vi "GLVT-Main_SingleLoop.vi"() -> ()   [LabVIEW 2020]
uses:
  Controls/GLVT-Stepper-EnableState.ctl
  Controls/GLVT-FlowmeterBankSelection.ctl
  Controls/GLVT-States.ctl
  Controls/GLVT-FGV-States.ctl
  Controls/GLVT-Stepper-RotateDirection.ctl
panel:
  in  "Flowmeter Bank":T1
  in  "Data Measure Time":dbl=1.0 min=1.0 step=0.1 format="%<%H:%M:%S>t"
  in  "Stop Button":bool
  out "Filename DTS":string
  out "Save Data Location":path
  in  "Filename Descriptor":string
  out "End Data Collection":bool
  out "Current Angle Array Location":i32
  out "Working":bool
  in  "Measure Valve Button":bool
  out "Collected Data":cluster{dbl[], dbl[]}(graph)
  out "Angles for Data Collection (deg abs)":dbl[](array[numeric])
  in  "Angle per Step":dbl=1.0 min=1.0 step=0.1
  in  "Max Angle to Rotate (deg abs)":dbl
  in  "Pulse Rate (pps)":i32=600
  in  "Steps per Rev":i32=1600
  in  "Move Stepper Button":bool
  in  "Angle to Rotate  (deg abs)":dbl step=0.1
  out "Motor Position Actual":dbl format="%#.2f"
  in  "Release Motor Button":bool
  in  "Motor State":T2
  # "Configuration Only\nDo Not Change"
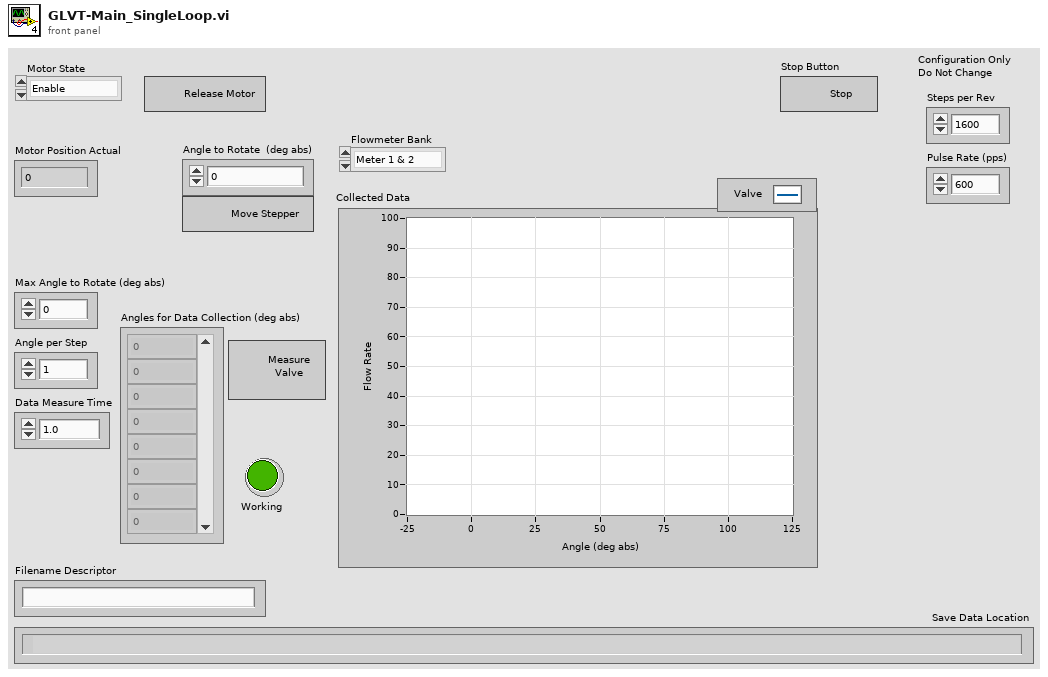
[diagram p1: front panel]
types:
  T1 = typedef "GLVT-FlowmeterBankSelection.ctl" = enum16{"Meter 1 & 2", "Meter 3 & 4", "Meter 5 & 6"}
  T2 = typedef "GLVT-Stepper-EnableState.ctl" = enum16{"Enable", "Disable"}
  T3 = typedef "GLVT-States.ctl" = enum16{"Idle", "Initialize", "Read Data", "Next Valve Pos", "Rotate Valve", "Save Data", "Exit"}
  T4 = typedef "GLVT-FGV-States.ctl" = enum16{"Get", "Set"}
  T5 = typedef "GLVT-Stepper-RotateDirection.ctl" = enum16{"CCW", "CW"}
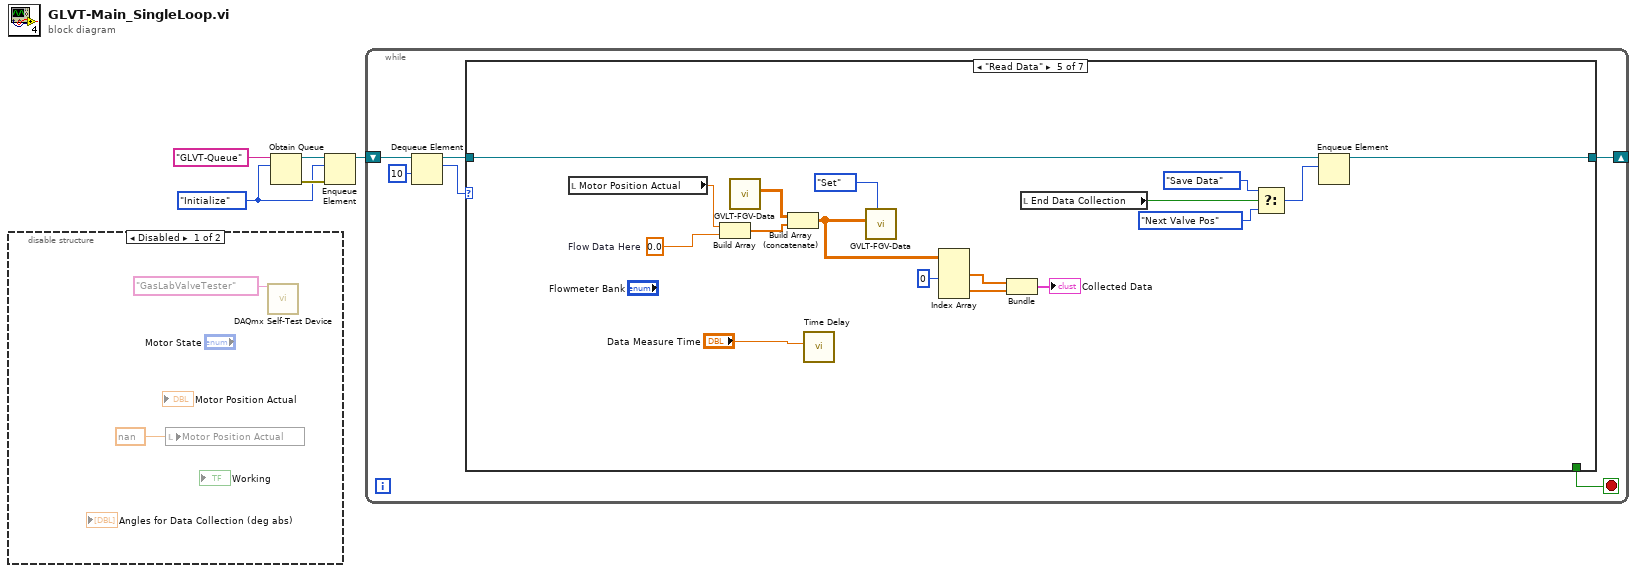
[diagram p0: block diagram]
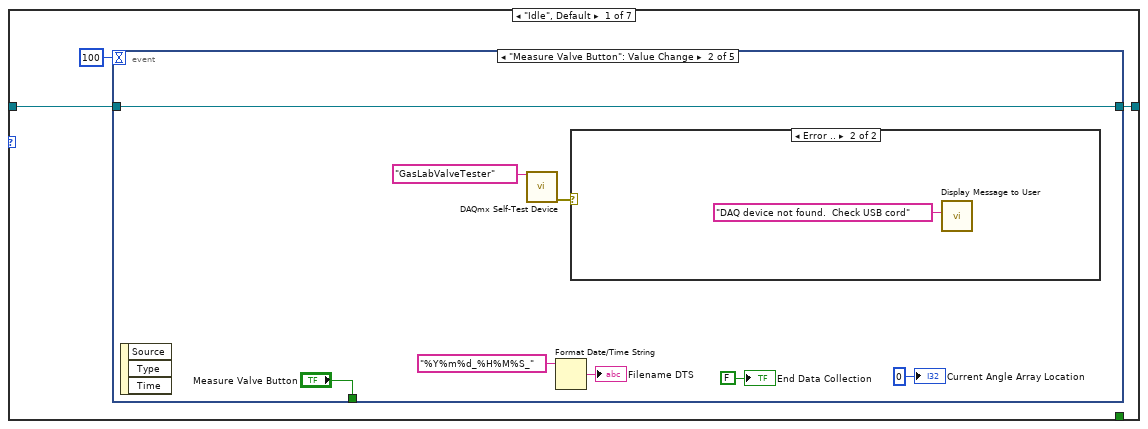
[diagram p2: hidden frame]
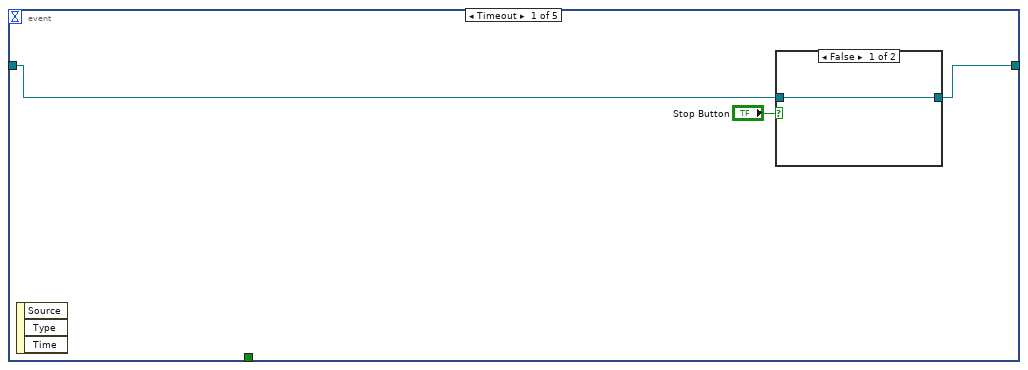
[diagram p3: hidden frame]
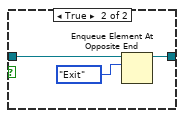
[diagram p4: hidden frame]
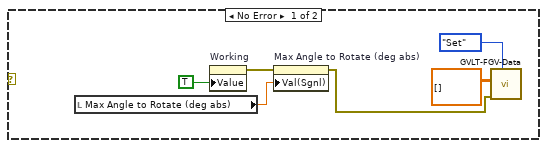
[diagram p5: hidden frame]
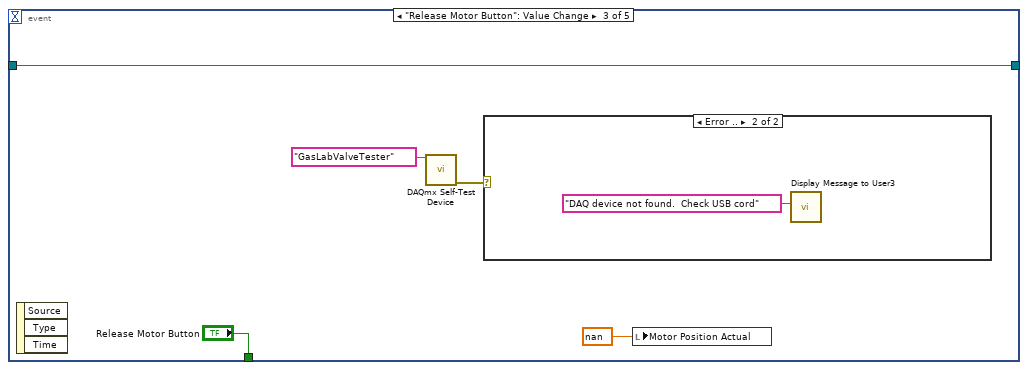
[diagram p6: hidden frame]
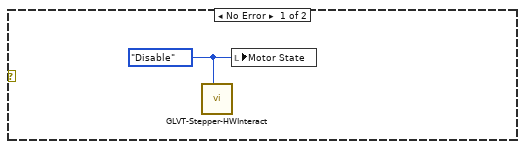
[diagram p7: hidden frame]
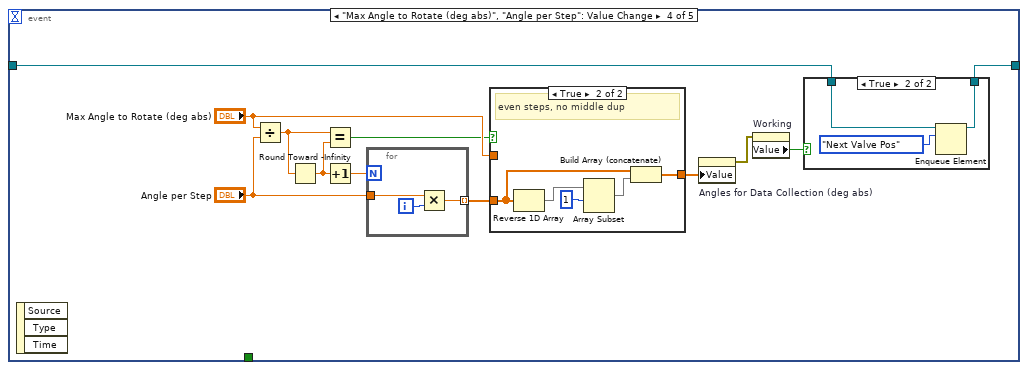
[diagram p8: hidden frame]
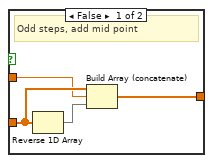
[diagram p10: hidden frame]
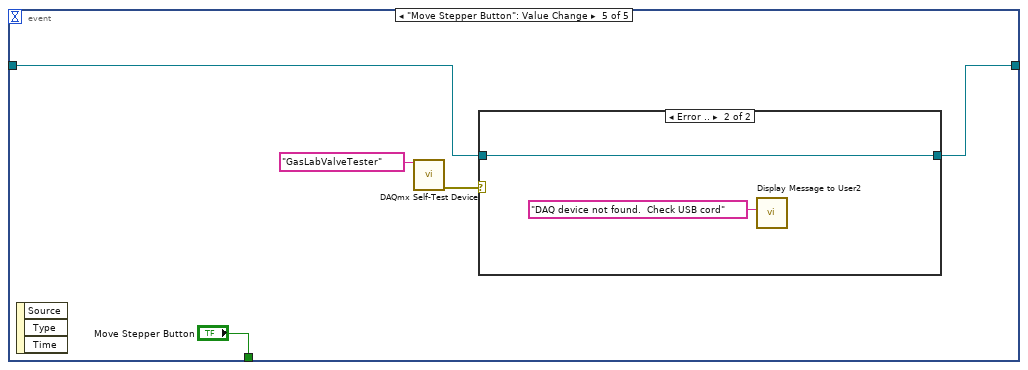
[diagram p11: hidden frame]
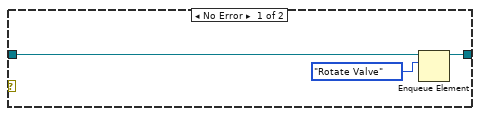
[diagram p12: hidden frame]
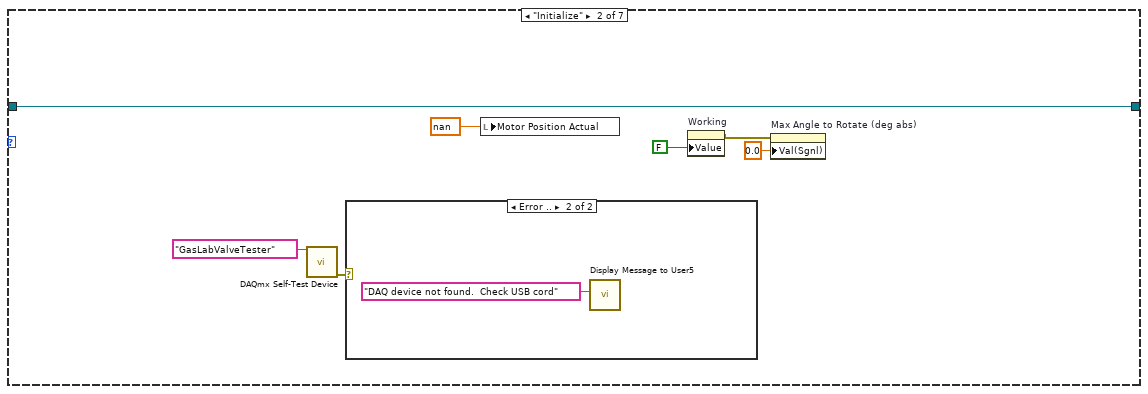
[diagram p13: hidden frame]
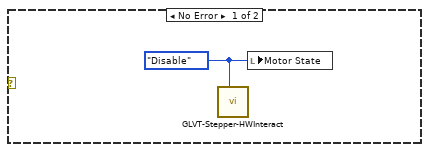
[diagram p14: hidden frame]
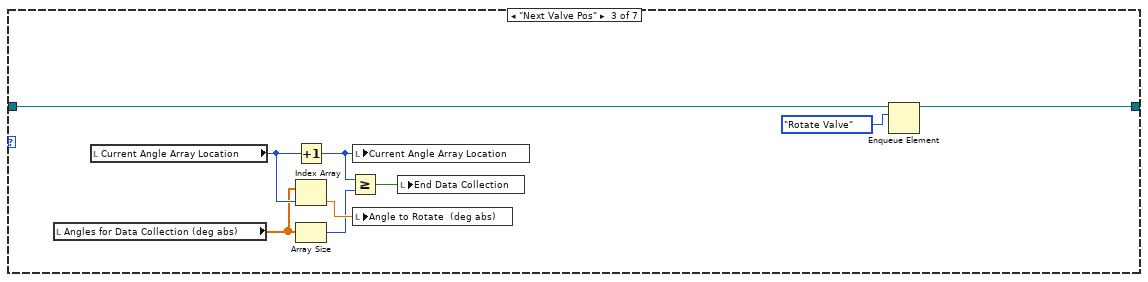
[diagram p15: hidden frame]
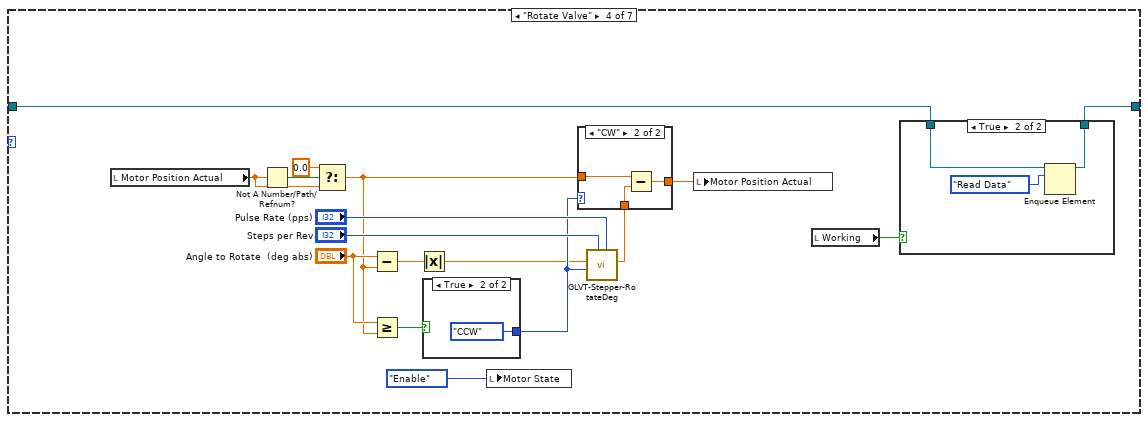
[diagram p16: hidden frame]
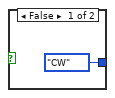
[diagram p18: hidden frame]
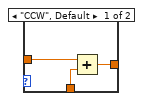
[diagram p19: hidden frame]
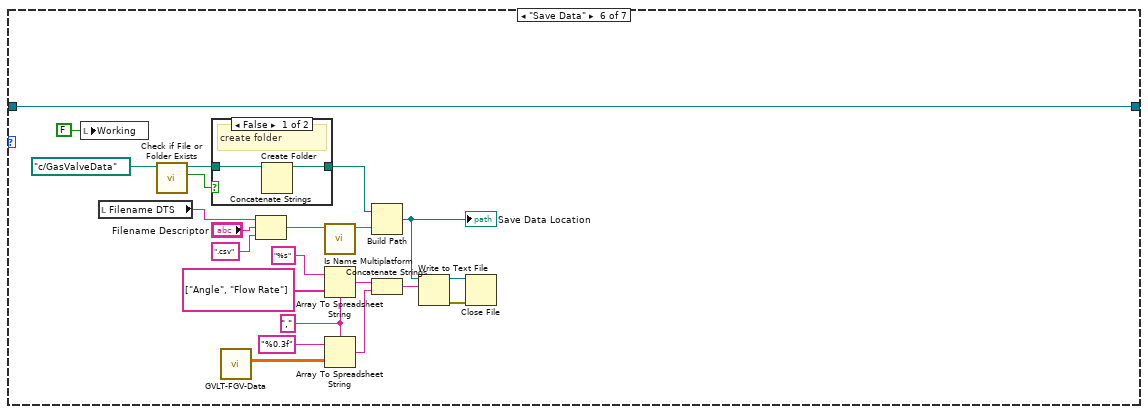
[diagram p20: hidden frame]
diagram:
  w2 = GLVT-States."Initialize"
  n1 = disable-structure shown="Disabled" {
    frame Disabled {
      n2 = local write "Motor Position Actual"(nan ("Motor Position")) -> ()
      n3 = call <vilib>:"DAQmx Self-Test Device.vi"("device in"=tag "GasLabValveTester") -> ()  [unwired: 14 in, 1 out]
    }
    frame Enabled {
    }
  }
  n4 = Obtain Queue(name (unnamed)="GLVT-Queue", element data type=w2) -> (queue out=w3:refnum<queue>, error out=w4:errorcluster)  [unwired: 3 in, 1 out]
  n5 = Enqueue Element(queue=w3, element=w2, error in (no error)=w4) -> (queue out=w1:refnum<queue>)  [unwired: 1 in, 2 out]
  n6 = while {
    shift-right: [w9] -> _
    shift-left: w1 -> [w12]
    stop <- w13 stop-if-true
    n7 = Dequeue Element(queue=w12, timeout in ms (-1)=10) -> (queue out=w11:refnum<queue>, element=w10:T3)  [unwired: 1 in, 2 out]
    n8 = case shown="\"Read Data\"" w10 {
      tunnel: [_ _ _ _ _ _ TRUE] -> w13
      tunnel: w11 -> [w15 w90 w101 w103 w147 w169 w177]
      tunnel: [w14 w90 w94 w102 w146 w169 w177] -> w9
      frame "Idle", Default {
        n9 = event shown="[1] \"Measure Valve Button\": Value Change" {
          selector: _ -> [_ _ _ _ _]
          dyn-events: _ -> [_ _ _ _ _]
          timeout: 100 -> [_ _ _ _ _]
          tunnel: w15 -> [w18 w31 w43 w47 w78]
          tunnel: [w19 w31 w43 w46 w76] -> w14
          tunnel: [_ "Measure Valve Button" "Release Motor Button" _ "Move Stepper Button"] -> _
          event Timeout {
            n10 = event-data() -> ()  [unwired: 1 in, 3 out]
            n11 = case shown="False" "Stop Button" {
              tunnel: [w20 w22] -> w19
              tunnel: w18 -> [w20 w21]
              frame False {
              }
              frame True {
                n12 = Enqueue Element At Opposite End(queue=w21, element=GLVT-States."Exit") -> (queue out=w22:refnum<queue>)  [unwired: 2 in, 2 out]
              }
            }
          }
          event "Measure Valve Button": Value Change {
            n13 = event-data() -> ()  [unwired: 1 in, 3 out]
            n14 = call <vilib>:"DAQmx Self-Test Device.vi"("device in"=tag "GasLabValveTester") -> ("error out"=w24:errorcluster)  [unwired: 14 in]
            n15 = Format Date/Time String(time format string (%c)="%Y%m%d_%H%M%S_") -> (date/time string=→"Filename DTS":string)  [unwired: 2 in]
            n16 = case shown="Error .." w24 {
              frame No Error {
                n17 = local read "Max Angle to Rotate (deg abs)"() -> (w37:dbl)
                n18 = property on="Working" class="Bool (strict)"("Value"=TRUE ("Working")) -> (error out=w35:errorcluster)  [unwired: 2 in, 1 out]
                n19 = property on="Max Angle to Rotate (deg abs)" class="DigNum (strict)"(error in=w35, "Val(Sgnl)"=w37) -> (error out=w32:errorcluster)  [unwired: 1 in, 1 out]
                n20 = call "GVLT-FGV-Data.vi"("State"=GLVT-FGV-States."Set", "error in"=w32, "Data In"=dbl[][] []) -> ()  [unwired: 7 in, 2 out]
              }
              frame Error {
                n21 = call "Display Message to User"("Message"="DAQ device not found.  Check USB cord") -> ()  [unwired: 9 in, 2 out]
              }
            }
            "Current Angle Array Location" <- 0 ("Current Angle Array Location")
            "End Data Collection" <- FALSE ("End Data Collection")
          }
          event "Release Motor Button": Value Change {
            n22 = event-data() -> ()  [unwired: 1 in, 3 out]
            n23 = call <vilib>:"DAQmx Self-Test Device.vi"("device in"=tag "GasLabValveTester") -> ("error out"=w39:errorcluster)  [unwired: 14 in]
            n24 = case shown="Error .." w39 {
              frame No Error {
                w44 = GLVT-Stepper-EnableState."Disable" ("GLVT-Enable State")
                n25 = call "GLVT-Stepper-HWInteract.vi"("GLVT-Enable State"=w44) -> ()  [unwired: 10 in, 1 out]
                n26 = local write "Motor State"(w44) -> ()
              }
              frame Error {
                n27 = call "Display Message to User3"("Message"="DAQ device not found.  Check USB cord") -> ()  [unwired: 9 in, 2 out]
              }
            }
            n28 = local write "Motor Position Actual"(nan ("Motor Position")) -> ()
          }
          event "Max Angle to Rotate (deg abs)", "Angle per Step": Value Change {
            n29 = event-data() -> ()  [unwired: 1 in, 3 out]
            n30 = Divide(x="Max Angle to Rotate (deg abs)", y="Angle per Step") -> (x/y=w53:dbl)
            n31 = Round Toward -Infinity(1:w53) -> (0:w52:dbl)
            n32 = Equal?(x=w53, y=w52) -> (x = y?=w51:bool)
            n33 = Increment(x=w52) -> (x+1=w57:dbl)
            n34 = for {
              N: w57 -> [_]
              tunnel: "Angle per Step" -> [w72]
              tunnel: [w71] -> w55 mode=indexing
              i -> [w73]
              n35 = Multiply(x=w72, y=w73) -> (x*y=w71:dbl)
            }
            n36 = case shown="True" w51 {
              tunnel: [w65 w66] -> w50
              tunnel: w55 -> [w64 w67]
              tunnel: "Max Angle to Rotate (deg abs)" -> [w62 _]
              frame False {
                # "Odd steps, add mid point"
                n37 = Reverse 1D Array(array=w64) -> (reversed array=w63:dbl[])
                n38 = Build Array (concatenate)(w64, w62, w63) -> (w65:dbl[])
              }
              frame True {
                # "even steps, no middle dup"
                n39 = Reverse 1D Array(array=w67) -> (reversed array=w70:dbl[])
                n40 = Array Subset(array=w70, index=1) -> (w68:dbl[])  [unwired: 1 in]
                n41 = Build Array (concatenate)(w67, w68) -> (w66:dbl[])
              }
            }
            n42 = property on="Angles for Data Collection (deg abs)" class="Arr (strict)"("Value"=w50) -> (error out=w49:errorcluster)  [unwired: 2 in, 1 out]
            n43 = property on="Working" class="Bool (strict)"(error in=w49) -> ("Value"=w48:bool)  [unwired: 1 in, 2 out]
            n44 = case shown="True" w48 {
              tunnel: [w58 w60] -> w46
              tunnel: w47 -> [w58 w61]
              frame False {
              }
              frame True {
                n45 = Enqueue Element(queue=w61, element=GLVT-States."Next Valve Pos") -> (queue out=w60:refnum<queue>)  [unwired: 2 in, 2 out]
              }
            }
          }
          event "Move Stepper Button": Value Change {
            n46 = event-data() -> ()  [unwired: 1 in, 3 out]
            n47 = call <vilib>:"DAQmx Self-Test Device.vi"("device in"=tag "GasLabValveTester") -> ("error out"=w74:errorcluster)  [unwired: 14 in]
            n48 = case shown="Error .." w74 {
              tunnel: w78 -> [w81 w83]
              tunnel: [w80 w83] -> w76
              frame No Error {
                n49 = Enqueue Element(queue=w81, element=GLVT-States."Rotate Valve") -> (queue out=w80:refnum<queue>)  [unwired: 2 in, 2 out]
              }
              frame Error {
                n50 = call "Display Message to User2"("Message"="DAQ device not found.  Check USB cord") -> ()  [unwired: 9 in, 2 out]
              }
            }
          }
        }
      }
      frame "Initialize" {
        n51 = call <vilib>:"DAQmx Self-Test Device.vi"("device in"=tag "GasLabValveTester") -> ("error out"=w84:errorcluster)  [unwired: 14 in]
        n52 = case shown="Error .." w84 {
          frame No Error {
            w91 = GLVT-Stepper-EnableState."Disable" ("GLVT-Enable State")
            n53 = call "GLVT-Stepper-HWInteract.vi"("GLVT-Enable State"=w91) -> ()  [unwired: 10 in, 1 out]
            n54 = local write "Motor State"(w91) -> ()
          }
          frame Error {
            n55 = call "Display Message to User5"("Message"="DAQ device not found.  Check USB cord") -> ()  [unwired: 9 in, 2 out]
          }
        }
        n56 = local write "Motor Position Actual"(nan ("Motor Position")) -> ()
        n57 = property on="Working" class="Bool (strict)"("Value"=FALSE ("Working")) -> (error out=w86:errorcluster)  [unwired: 2 in, 1 out]
        n58 = property on="Max Angle to Rotate (deg abs)" class="DigNum (strict)"(error in=w86, "Val(Sgnl)"=0.0 ("Value (Signaling)")) -> ()  [unwired: 1 in, 2 out]
      }
      frame "Next Valve Pos" {
        n59 = local read "Angles for Data Collection (deg abs)"() -> (w98:dbl[])
        n60 = local read "Current Angle Array Location"() -> (w100:i32)
        n61 = Increment(x=w100) -> (x+1=w96:i32)
        n62 = Index Array(array=w98, index=w100) -> (element=w99:dbl)
        n63 = Array Size(array=w98) -> (size(s)=w97:i32)
        n64 = Greater Or Equal?(x=w96, y=w97) -> (x >= y?=w95:bool)
        n65 = local write "Current Angle Array Location"(w96) -> ()
        n66 = local write "Angle to Rotate  (deg abs)"(w99) -> ()
        n67 = local write "End Data Collection"(w95) -> ()
        n68 = Enqueue Element(queue=w101, element=GLVT-States."Rotate Valve") -> (queue out=w94:refnum<queue>)  [unwired: 2 in, 2 out]
      }
      frame "Rotate Valve" {
        n69 = local read "Motor Position Actual"() -> (w112:dbl)
        n70 = Not A Number/Path/Refnum?(number/path/refnum=w112) -> (NaN/Path/Refnum?=w113:bool)
        n71 = Select(t=0.0, s=w113, f=w112) -> (s? t:f=w108:dbl)
        n72 = Subtract(x="Angle to Rotate  (deg abs)", y=w108) -> (x-y=w107:dbl)
        n73 = Greater Or Equal?(x="Angle to Rotate  (deg abs)", y=w108) -> (x >= y?=w111:bool)
        n74 = Absolute Value(x=w107) -> (abs(x)=w106:dbl)
        n75 = case shown="True" w111 {
          tunnel: [GLVT-Stepper-RotateDirection."CW" ("Rotate Direction") GLVT-Stepper-RotateDirection."CCW" ("Rotate Direction")] -> w110
          frame False {
          }
          frame True {
          }
        }
        n76 = local write "Motor State"(GLVT-Stepper-EnableState."Enable" ("GLVT-Enable State")) -> ()
        n77 = call "GLVT-Stepper-RotateDeg.vi"("Pulse Rate (pps)"="Pulse Rate (pps)", "Steps per Rev"="Steps per Rev", "Rotate Direction"=w110, "Rotation Angle (deg)"=w106) -> ("Actual Rotation Angle (deg)"=w118:dbl)  [unwired: 6 in, 1 out]
        n78 = case shown="\"CW\"" w110 {
          tunnel: w108 -> [w127 w130]
          tunnel: w118 -> [w126 w129]
          tunnel: [w125 w128] -> w105
          frame "CCW", Default {
            n79 = Add(x=w127, y=w126) -> (x+y=w125:dbl)
          }
          frame "CW" {
            n80 = Subtract(x=w130, y=w129) -> (x-y=w128:dbl)
          }
        }
        n81 = local write "Motor Position Actual"(w105) -> ()
        n82 = local read "Working"() -> (w104:bool)
        n83 = case shown="True" w104 {
          tunnel: [w119 w121] -> w102
          tunnel: w103 -> [w119 w122]
          frame False {
          }
          frame True {
            n84 = Enqueue Element(queue=w122, element=GLVT-States."Read Data") -> (queue out=w121:refnum<queue>)  [unwired: 2 in, 2 out]
          }
        }
      }
      frame "Read Data" {
        w131 = 0.0  # Flow Data Here
        n85 = local read "Motor Position Actual"() -> (w141:dbl)
        n86 = Build Array(w141, w131) -> (w139:dbl[])
        n87 = call "GVLT-FGV-Data.vi"() -> ("Data Out"=w140:dbl[][])  [unwired: 10 in, 1 out]
        n88 = Build Array (concatenate)(w140, w139) -> (w137:dbl[][])
        n89 = call "Time Delay"("Delay Time (s)"="Data Measure Time") -> ()  [unwired: 10 in, 1 out]
        n90 = call "GVLT-FGV-Data.vi"("State"=GLVT-FGV-States."Set", "Data In"=w137) -> ()  [unwired: 8 in, 2 out]
        n91 = Index Array(array=w137, index (col) #1=0 ("disabled index (col)")) -> (element #1=w135:dbl[], element #2=w134:dbl[])  [unwired: 3 in]
        n92 = Bundle(w135, w134) -> (→"Collected Data":cluster{dbl[], dbl[]})  [unwired: 1 in]
        n93 = local read "End Data Collection"() -> (w145:bool)
        n94 = Select(t=GLVT-States."Save Data" ("element"), s=w145, f=GLVT-States."Next Valve Pos" ("element")) -> (s? t:f=w142:T3)
        n95 = Enqueue Element(queue=w147, element=w142) -> (queue out=w146:refnum<queue>)  [unwired: 2 in, 2 out]
      }
      frame "Save Data" {
        w157 = "," ("delimiter (Tab)")
        n96 = local write "Working"(FALSE ("Working")) -> ()
        n97 = local read "Filename DTS"() -> (w166:string)
        n98 = call <vilib>:"Check if File or Folder Exists.vi"("path"=path "c:/GasValveData") -> ("file or folder exists?"=w162:bool, "dup path"=w161:path)  [unwired: 8 in, 1 out]
        n99 = case shown="False" w162 {
          tunnel: w161 -> [w171 w172]
          tunnel: [w170 w172] -> w153
          frame False {
            # "create folder"
            n100 = Create Folder(path (use dialog)=w171) -> (created path=w170:path)  [unwired: 2 in, 2 out]
          }
          frame True {
            # "exists, do nothing"
          }
        }
        n101 = call "GVLT-FGV-Data.vi"() -> ("Data Out"=w160:dbl[][])  [unwired: 10 in, 1 out]
        n102 = Concatenate Strings(w166, "Filename Descriptor", ".csv" ("string")) -> (w164:string)
        n103 = call <vilib>:"Is Name Multiplatform.vi"("filename"=w164) -> ("suggested filename"=w152:string)  [unwired: 6 in, 4 out]
        n104 = Array To Spreadsheet String(delimiter (Tab)=w157, array=string[] ["Angle", "Flow Rate"], 3:"%s" ("format string")) -> (spreadsheet string=w155:string)
        n105 = Array To Spreadsheet String(delimiter (Tab)=w157, array=w160, 3:"%0.3f" ("format string")) -> (spreadsheet string=w154:string)
        n106 = Build Path(base path=w153, name or relative path=w152) -> (appended path=w148:path)
        "Save Data Location" <- w148
        n107 = Concatenate Strings(w155, w154) -> (w151:string)
        n108 = Write to Text File(file (use dialog)=w148, text=w151) -> (refnum out=w149:refnum<file>, error out=w150:errorcluster)  [unwired: 2 in, 1 out]
        n109 = Close File(refnum=w149, error in=w150) -> ()  [unwired: 2 out]
      }
      frame "Exit" {
        n110 = local write "Motor Position Actual"(nan ("Motor Position")) -> ()
        n111 = local write "Working"(FALSE ("Working")) -> ()
        n112 = call <vilib>:"DAQmx Self-Test Device.vi"("device in"=tag "GasLabValveTester") -> ("error out"=w173:errorcluster)  [unwired: 14 in]
        n113 = case shown="Error .." w173 {
          frame No Error {
            w179 = GLVT-Stepper-EnableState."Disable" ("GLVT-Enable State")
            n114 = call "GLVT-Stepper-HWInteract.vi"("GLVT-Enable State"=w179) -> ()  [unwired: 10 in, 1 out]
            n115 = local write "Motor State"(w179) -> ()
          }
          frame Error {
            n116 = call "Display Message to User4"("Message"="DAQ device not found.  Verify that the DAQ is off and safe.") -> ()  [unwired: 9 in, 2 out]
          }
        }
      }
    }
  }
